vi "Control Pressure Regulator.vi"(4 "Timeout":i32=30, 8 "error in":errorcluster, 11 "Desired PSI":dbl) -> (0 "error out":errorcluster, 3 "Reached Setpoint?":bool)   [LabVIEW 2015]
panel:
  out "NI-DAQ Pressure":dbl
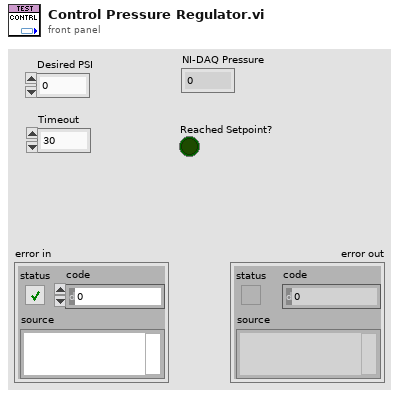
[diagram p1: front panel]
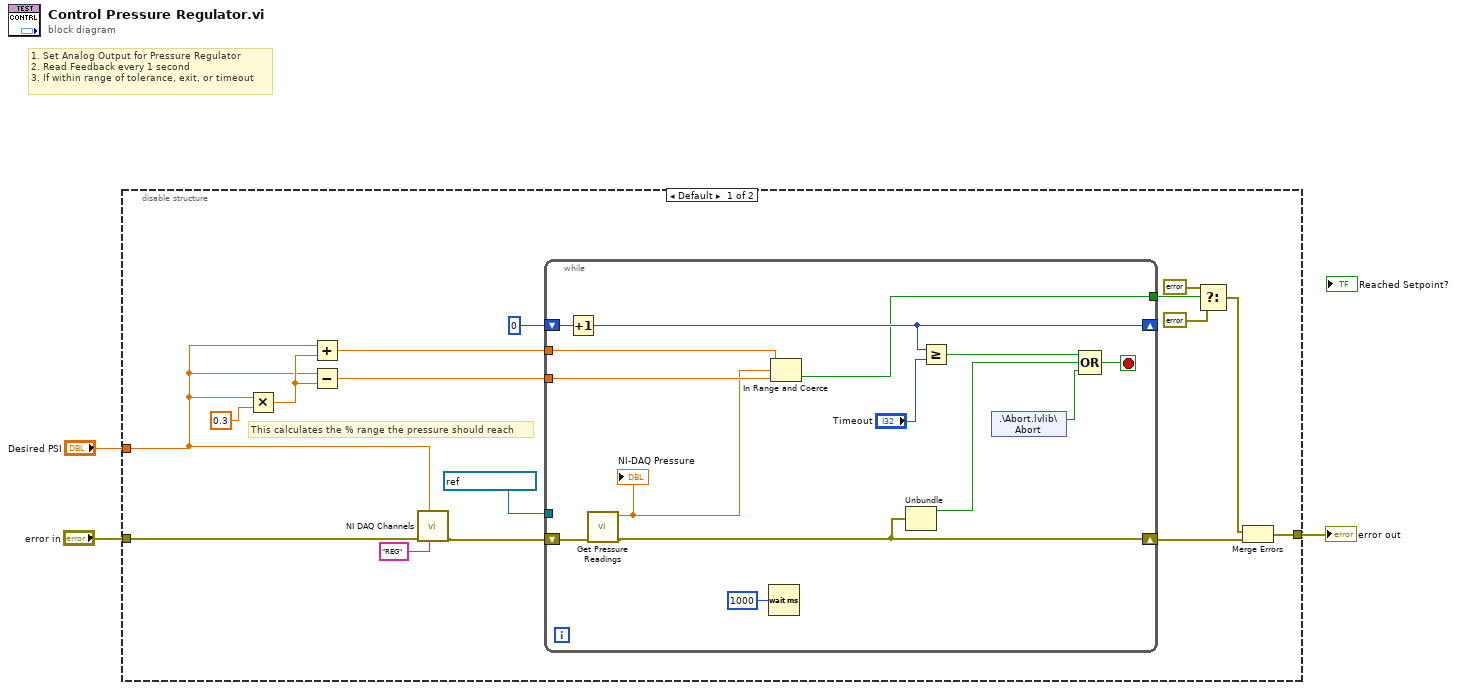
[diagram p0: block diagram]
diagram:
  # "1. Set Analog Output for Pressure Regulator\n2. Read Feedback every 1 second\n3. If within range of tolerance, exit, or timeout"
  n1 = disable-structure shown="Default" {
    disable-tunnel: "error in" -> [w7 w34]
    disable-tunnel: "Desired PSI" -> [w4 _]
    disable-tunnel: [w12 w34] -> w1
    frame condition #0 (active) {
      # "This calculates the % range the pressure should reach"
      n2 = Multiply(x=w4, y=0.3) -> (x*y=w8:dbl)
      n3 = Add(x=w4, y=w8) -> (x+y=w9:dbl)
      n4 = Subtract(x=w4, y=w8) -> (x-y=w17:dbl)
      n5 = call "NI DAQ Channels.vi"("Channel"="REG", "AO Data"=w4, "error in (no error)"=w7) -> ("error out"=w6:errorcluster)  [unwired: 7 in, 1 out]
      n6 = while {
        tunnel: refnum<k21> "Pressure_GC" -> [_]
        shift-right: [w22] -> w14
        shift-left: w6 -> [w23]
        tunnel: w17 -> [w32]
        tunnel: w9 -> [w33]
        shift-right: [w28] -> _
        shift-left: 0 -> [w29]
        tunnel: [w20] -> w15
        stop <- w30 stop-if-true
        n7 = Increment(x=w29) -> (x+1=w28:i32)
        n8 = call "Get Pressure Readings.vi"("error in (no error)"=w23) -> ("error out"=w22:errorcluster, "NI-DAQ Pressure"=w21:dbl)  [unwired: 6 in, 3 out]
        "NI-DAQ Pressure" <- w21
        n9 = Wait (ms)(milliseconds to wait=u32 1000) -> ()  [unwired: 1 out]
        n10 = In Range and Coerce(upper limit=w33, x=w21, lower limit=w32) -> (In Range?=w20:bool)  [unwired: 1 out]
        n11 = Unbundle(w22) -> ("status"=w31:bool)  [unwired: 2 out]
        n12 = Greater Or Equal?(x=w28, y="Timeout") -> (x >= y?=w24:bool)
        n13 = shared-variable ".\\Abort.lvlib\\Abort"() -> (w26:bool)  [unwired: 1 in, 1 out]
        n14 = Compound Arithmetic op=OR(w24, w31, w26) -> (w30:bool)
      }
      n15 = Select(t=errorcluster {"status"=FALSE, "code"=0, "source"=""} ("error out"), s=w15, f=errorcluster {"status"=TRUE, "code"=9000, "source"="Timeout Error. Pressure Regulator Failed to Reach Setpoint"} ("error out")) -> (s? t:f=w13:errorcluster)
      n16 = Merge Errors(w13, w14) -> (w12:errorcluster)
    }
    frame condition #1 {
    }
  }
  "error out" <- w1
